vi "INI_Write Data To LabVIEW INI.vi"(8 "error in (no error)":errorcluster, 11 "INI Data":T1={"Show Layer Tab?"=FALSE, "Show Terminals?"=FALSE, "Text"={"Font"="", "Alignment"=0, "Size"=0}, "3rd party Templates"={"Store 3rd party Templates?"=FALSE, "Folder Name"=""}, "Merge user layers on commit"=FALSE, "Body Text"={"Line 1 text"="", "Line 2 text"="", "Line 3 text"="", "Line 4 text"="", "Line 1 color"=0, "Line 2 color"=0, "Line 3 color"=0, "Line 4 color"=0, "Body Text Spec"={"Font"="", "Alignment"=0, "Size"=3}, "Center text vertically"=FALSE, "Capitalize Text"=FALSE}, "Fill Color"=0, "Edge Color"=0, "Tab"=0, "Tool"=enum."Ellipse", "Disable Layers?"=FALSE} {"Body Text"."Body Text Spec"."Alignment" items=["left", "center", "right"]; "Text"."Alignment" items=["left", "center", "right"]}) -> (0 "error out":errorcluster)   [LabVIEW 2021]
uses:
  TypeDefs/Cluster_INI Data.ctl
  vi.lib/LabVIEW Icon API/lv_icon/Controls/Font.ctl
  vi.lib/LabVIEW Icon API/lv_icon/Controls/Alignment.ctl
  TypeDefs/Num_Font Size.ctl
  TypeDefs/Cluster_BodyText.ctl
  vi.lib/LabVIEW Icon API/lv_icon/Controls/IEColor.ctl
  TypeDefs/Cluster_Button Draw Tools.ctl
  TypeDefs/Bool_Draw Tool.ctl
  TypeDefs/Bool_Line Tool.ctl
  TypeDefs/Bool_ColorExtractor Tool.ctl
  TypeDefs/Bool_Fill Tool.ctl
  TypeDefs/Bool_IERect Tool.ctl
  TypeDefs/Bool_FRect Tool.ctl
  TypeDefs/Bool_Circle Tool.ctl
  TypeDefs/Bool_FillCircle Tool.ctl
  TypeDefs/Bool_Eraser Tool.ctl
  TypeDefs/Bool_Text Tool.ctl
  TypeDefs/Bool_Selection Tool.ctl
  TypeDefs/Bool_Move Tool.ctl
  <resource>/dialog/lvconfig.llb/LV Config Write String.vi
  <resource>/dialog/lvconfig.llb/LV Config Write Color.vi
  <resource>/dialog/lvconfig.llb/LV Config Write Boolean.vi
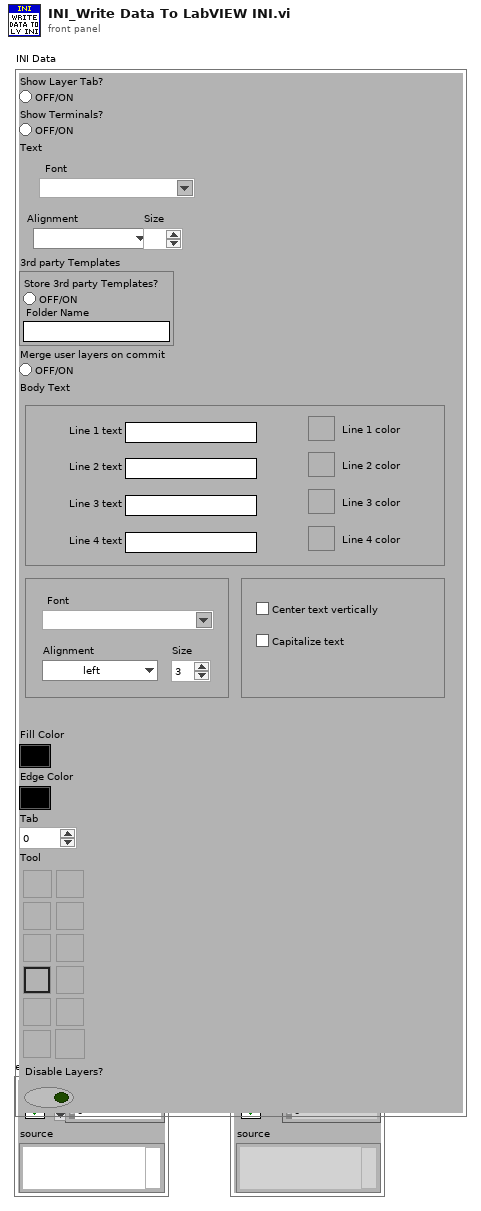
[diagram p1: front panel]
types:
  T1 = typedef "Cluster_INI Data.ctl" = cluster{"Show Layer Tab?":bool, "Show Terminals?":bool, "Text":cluster{"Font":T2, "Alignment":T3, "Size":T4}, "3rd party Templates":cluster{"Store 3rd party Templates?":bool, "Folder Name":string}, "Merge user layers on commit":bool, "Body Text":T5, "Fill Color":T6, "Edge Color":T6, "Tab":u16, "Tool":T7, "Disable Layers?":bool}
  T2 = typedef "Font.ctl" = string
  T3 = typedef "Alignment.ctl" = u16
  T4 = typedef "Num_Font Size.ctl" = u8
  T5 = typedef "Cluster_BodyText.ctl" = cluster{"Line 1 text":string, "Line 2 text":string, "Line 3 text":string, "Line 4 text":string, "Line 1 color":u32, "Line 2 color":u32, "Line 3 color":u32, "Line 4 color":u32, "Body Text Spec":cluster{"Font":T2, "Alignment":T3, "Size":u8}, "Center text vertically":bool, "Capitalize Text":bool}
  T6 = typedef "IEColor.ctl" = u32
  T7 = typedef "Cluster_Button Draw Tools.ctl" = enum32{"Pencil", "Line", "Dropper", "Fill", "Rectangle", "Filled Rectangle", "Ellipse", "Filled Ellipse", "Eraser", "Text", "Select", "Move"}
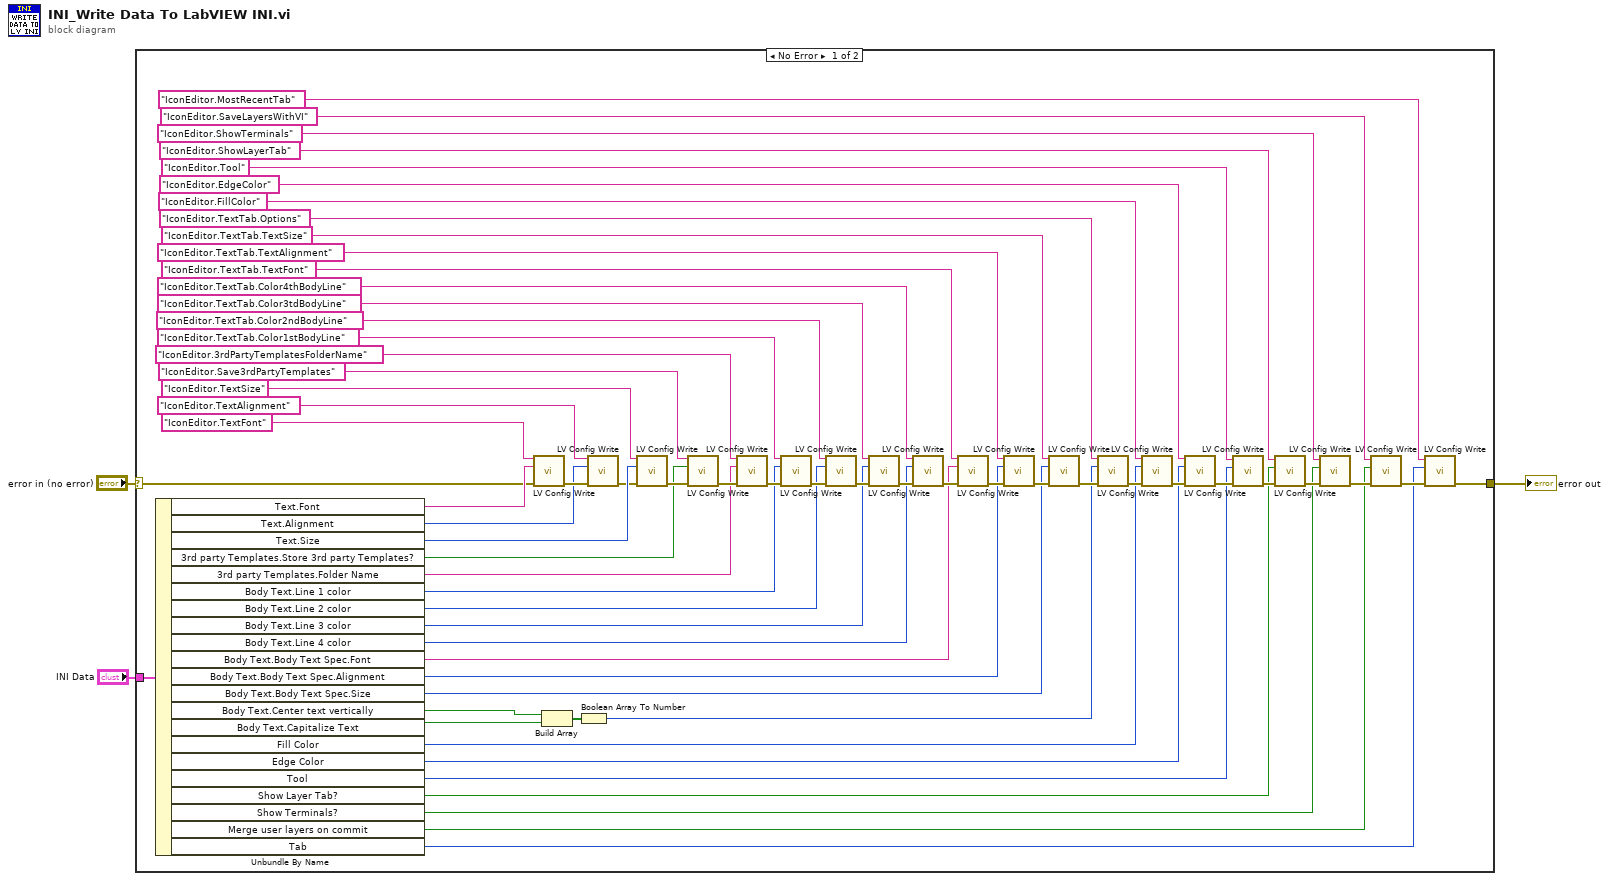
[diagram p0: block diagram]
diagram:
  n1 = case shown="No Error" "error in (no error)" {
    selector: "error in (no error)" -> [w5 w69]
    tunnel: [w4 w69] -> w2
    tunnel: "INI Data" -> [w68 _]
    frame No Error {
      n2 = Unbundle By Name(w68) -> ("Text.Font"=w67:T2, "Text.Alignment"=w64:T3, "Text.Size"=w62:T4, "3rd party Templates.Store 3rd party Templates?"=w58:bool, "3rd party Templates.Folder Name"=w55:string, "Body Text.Line 1 color"=w47:u32, "Body Text.Line 2 color"=w46:u32, "Body Text.Line 3 color"=w43:u32, "Body Text.Line 4 color"=w42:u32, "Body Text.Body Text Spec.Font"=w38:T2, "Body Text.Body Text Spec.Alignment"=w37:T3, "Body Text.Body Text Spec.Size"=w36:u8, "Body Text.Center text vertically"=w31:bool, "Body Text.Capitalize Text"=w32:bool, "Fill Color"=w22:T6, "Edge Color"=w21:T6, "Tool"=w18:T7, "Show Layer Tab?"=w15:bool, "Show Terminals?"=w14:bool, "Merge user layers on commit"=w9:bool, "Tab"=w6:u16)
      n3 = call-poly <resource>:"LV Config Write.vi"("error in (no error)"=w5, "value"=w67, "key"="IconEditor.TextFont") -> ("error out"=w65:errorcluster)  [unwired: 4 out]
      n4 = Build Array(w31, w32) -> (w30:bool[])
      n5 = Boolean Array To Number(Boolean array=w30) -> (number=w27:u32)
      n6 = call-poly <resource>:"LV Config Write.vi"("error in (no error)"=w65, "value"=w64, "key"="IconEditor.TextAlignment") -> ("error out"=w61:errorcluster)  [unwired: 4 out]
      n7 = call-poly <resource>:"LV Config Write.vi"("error in (no error)"=w61, "value"=w62, "key"="IconEditor.TextSize") -> ("error out"=w59:errorcluster)  [unwired: 4 out]
      n8 = call-poly <resource>:"LV Config Write.vi"("error in (no error)"=w59, "value"=w58, "key"="IconEditor.Save3rdPartyTemplates") -> ("error out"=w56:errorcluster)  [unwired: 4 out]
      n9 = call-poly <resource>:"LV Config Write.vi"("error in (no error)"=w56, "value"=w55, "key"="IconEditor.3rdPartyTemplatesFolderName") -> ("error out"=w53:errorcluster)  [unwired: 4 out]
      n10 = call-poly <resource>:"LV Config Write.vi"("error in (no error)"=w53, "value"=w47, "key"="IconEditor.TextTab.Color1stBodyLine") -> ("error out"=w52:errorcluster)  [unwired: 4 out]
      n11 = call-poly <resource>:"LV Config Write.vi"("error in (no error)"=w52, "value"=w46, "key"="IconEditor.TextTab.Color2ndBodyLine") -> ("error out"=w45:errorcluster)  [unwired: 4 out]
      n12 = call-poly <resource>:"LV Config Write.vi"("error in (no error)"=w45, "value"=w43, "key"="IconEditor.TextTab.Color3tdBodyLine") -> ("error out"=w44:errorcluster)  [unwired: 4 out]
      n13 = call-poly <resource>:"LV Config Write.vi"("error in (no error)"=w44, "value"=w42, "key"="IconEditor.TextTab.Color4thBodyLine") -> ("error out"=w41:errorcluster)  [unwired: 4 out]
      n14 = call-poly <resource>:"LV Config Write.vi"("error in (no error)"=w41, "value"=w38, "key"="IconEditor.TextTab.TextFont") -> ("error out"=w40:errorcluster)  [unwired: 4 out]
      n15 = call-poly <resource>:"LV Config Write.vi"("error in (no error)"=w40, "value"=w37, "key"="IconEditor.TextTab.TextAlignment") -> ("error out"=w39:errorcluster)  [unwired: 4 out]
      n16 = call-poly <resource>:"LV Config Write.vi"("error in (no error)"=w39, "value"=w36, "key"="IconEditor.TextTab.TextSize") -> ("error out"=w29:errorcluster)  [unwired: 4 out]
      n17 = call-poly <resource>:"LV Config Write.vi"("error in (no error)"=w29, "value"=w27, "key"="IconEditor.TextTab.Options") -> ("error out"=w26:errorcluster)  [unwired: 4 out]
      n18 = call-poly <resource>:"LV Config Write.vi"("error in (no error)"=w26, "value"=w22, "key"="IconEditor.FillColor") -> ("error out"=w25:errorcluster)  [unwired: 4 out]
      n19 = call-poly <resource>:"LV Config Write.vi"("error in (no error)"=w25, "value"=w21, "key"="IconEditor.EdgeColor") -> ("error out"=w20:errorcluster)  [unwired: 4 out]
      n20 = call-poly <resource>:"LV Config Write.vi"("error in (no error)"=w20, "value"=w18, "key"="IconEditor.Tool") -> ("error out"=w16:errorcluster)  [unwired: 4 out]
      n21 = call-poly <resource>:"LV Config Write.vi"("error in (no error)"=w16, "value"=w15, "key"="IconEditor.ShowLayerTab") -> ("error out"=w17:errorcluster)  [unwired: 4 out]
      n22 = call-poly <resource>:"LV Config Write.vi"("error in (no error)"=w17, "value"=w14, "key"="IconEditor.ShowTerminals") -> ("error out"=w11:errorcluster)  [unwired: 4 out]
      n23 = call-poly <resource>:"LV Config Write.vi"("error in (no error)"=w11, "value"=w9, "key"="IconEditor.SaveLayersWithVI") -> ("error out"=w8:errorcluster)  [unwired: 4 out]
      n24 = call-poly <resource>:"LV Config Write.vi"("error in (no error)"=w8, "value"=w6, "key"="IconEditor.MostRecentTab") -> ("error out"=w4:errorcluster)  [unwired: 4 out]
    }
    frame Error {
    }
  }
  "error out" <- w2
